vi "Set-exit.vi"(8 "error in (no error)":errorcluster, 10 "Exit":bool, 11 "Object ref in":T1) -> (0 "error out":errorcluster, 3 "Object ref out":T1)   [LabVIEW 2013, in "PowderDeposition.lvlib" / "PD-Main.lvclass"]
uses:
  PD-Main.lvclass
  Object-reference.ctl
  PD-Main.lvclass/PD-Main.ctl
  Read Exit.vi
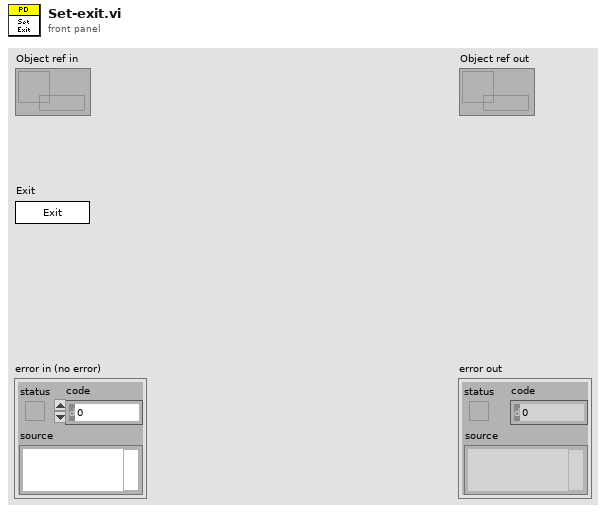
[diagram p1: front panel]
types:
  T1 = typedef "PowderDeposition.lvlib/PD-Main.lvclass/Object-reference.ctl" = refnum<data-value>
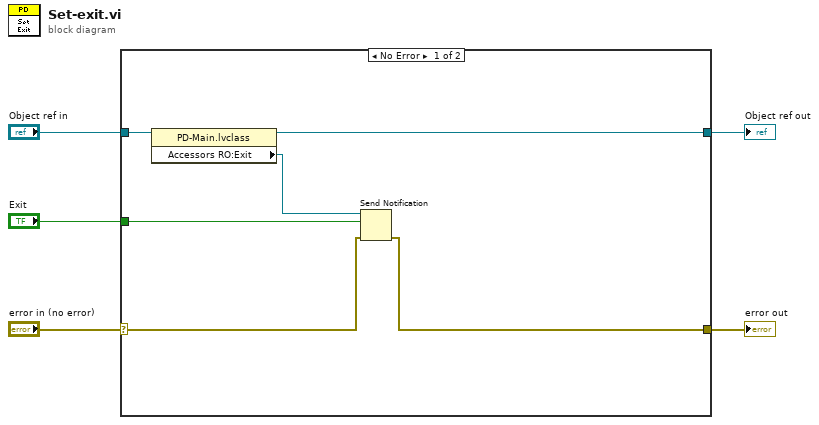
[diagram p0: block diagram]
diagram:
  n1 = case shown="No Error" "error in (no error)" {
    selector: "error in (no error)" -> [w7 w13]
    tunnel: [w6 w13] -> w4
    tunnel: [w10 w12] -> w2
    tunnel: "Object ref in" -> [w11 w12]
    tunnel: "Exit" -> [w8 _]
    frame No Error {
      n2 = property class="PD-Main.lvclass"(reference=w11) -> (reference out=w10:T1, "Accessors RO:Exit"=w9:refnum<notifier>)  [unwired: 1 in, 1 out]
      n3 = Send Notification(notification=w8, notifier=w9, error in (no error)=w7) -> (error out=w6:errorcluster)  [unwired: 1 out]
    }
    frame Error {
    }
  }
  "error out" <- w4
  "Object ref out" <- w2
